vi "_Read_C.vi"(8 "error in (no error)":errorcluster, 11 "Postgres Connector In":refnum<class "Postgres Connector.lvclass">) -> (0 "error out":errorcluster, 1 "Another Query?":bool, 2 "No return?":bool, 3 "Postgres Connector Out":refnum<class "Postgres Connector.lvclass">)   [LabVIEW 2020, in "Postgres Connector.lvclass"]
doc: "This VI decode the \"C\" section of the message sent by the database. It also check if a another query has been sent. It return the type of query that has been completed"
uses:
  Postgres Connector.lvclass
  Cluster_Reader_Infos.ctl
  Enum_RowDescription_State_Machine.ctl
  Postgres Connector.lvclass/Postgres Connector.ctl
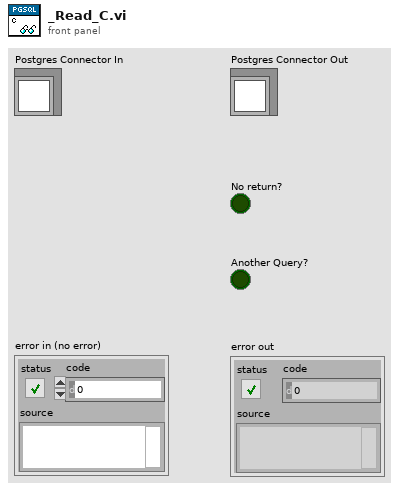
[diagram p1: front panel]
types:
  T1 = typedef "Postgres Connector.lvclass/Enum_RowDescription_State_Machine.ctl" = enum16{"Check For Error", "Wait For T", "Wait For D", "Wait For Z", "C Byte Length", "Z Byte Length", "n Byte Length", "Byte Length", "Get Infos", "Check For End", "Flush", "Quit"}
  T2 = typedef "Postgres Connector.lvclass/Cluster_Reader_Infos.ctl" = cluster{"Byte Length":i32}
  T3 = enum16{"Standard", "Buffered", "CRLF", "Immediate"}
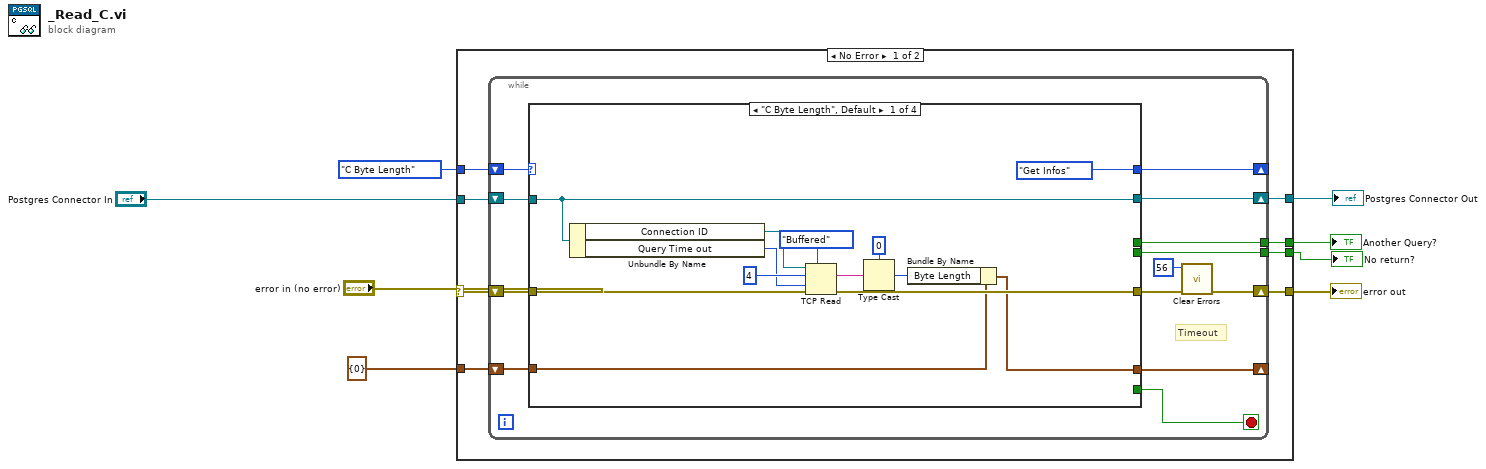
[diagram p0: block diagram]
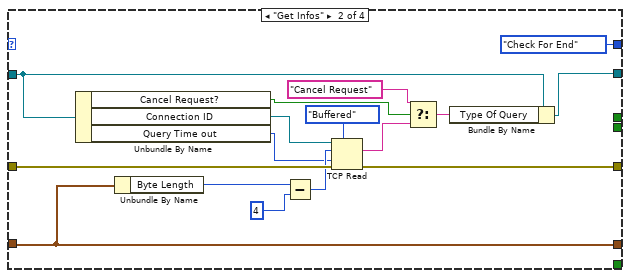
[diagram p2: hidden frame]
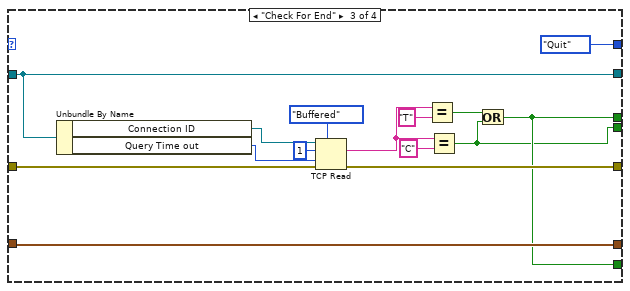
[diagram p3: hidden frame]
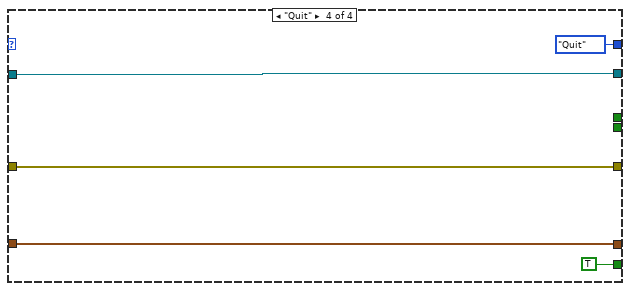
[diagram p4: hidden frame]
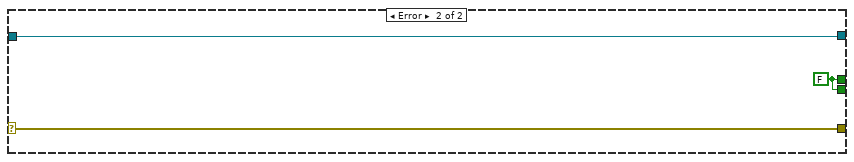
[diagram p5: hidden frame]
diagram:
  n1 = case shown="No Error" "error in (no error)" {
    selector: "error in (no error)" -> [w15 w81]
    tunnel: "Postgres Connector In" -> [w16 w80]
    tunnel: Enum_RowDescription_State_Machine."C Byte Length" -> [w14 _]
    tunnel: [w13 w81] -> w6
    tunnel: T2 {"Byte Length"=0} ("Reader_Infos") -> [w12 _]
    tunnel: [w11 w79] -> w4
    tunnel: [w10 w80] -> w3
    tunnel: [w9 w79] -> w2
    frame No Error {
      n2 = while {
        shift-right: [w25] -> w13
        shift-left: w15 -> [w28]
        shift-right: [w23] -> _
        shift-left: w14 -> [w27]
        shift-right: [w21] -> _
        shift-left: w12 -> [w22]
        tunnel: [w19] -> w11
        shift-right: [w18] -> w10
        shift-left: w16 -> [w29]
        tunnel: [w17] -> w9
        stop <- w20 stop-if-true
        # "Timeout"
        n3 = case shown="\"C Byte Length\", Default" w27 {
          tunnel: w29 -> [w38 w49 w65 w74]
          tunnel: w28 -> [w39 w56 w69 w77]
          tunnel: [w37 w55 w68 w77] -> w26
          tunnel: [Enum_RowDescription_State_Machine."Get Infos" Enum_RowDescription_State_Machine."Check For End" Enum_RowDescription_State_Machine."Quit" Enum_RowDescription_State_Machine."Quit"] -> w23
          tunnel: w22 -> [w36 w53 w67 w78]
          tunnel: [w35 w53 w67 w78] -> w21
          tunnel: [_ _ w62 TRUE] -> w20
          tunnel: [_ _ w62 _] -> w19
          tunnel: [w38 w48 w65 w74] -> w18
          tunnel: [_ _ w61 _] -> w17
          frame "C Byte Length", Default {
            n4 = Unbundle By Name(w38) -> ("Connection ID"=w41:refnum<k5>, "Query Time out"=w30:i32)
            n5 = TCP Read(connection ID=w41, bytes to read=4, error in (no error)=w39, 7:T3."Buffered" ("mode (standard)"), 9:w30) -> (data out=w31:string, error out=w37:errorcluster)  [unwired: 1 out]
            n6 = Type Cast(type=0, x=w31) -> (*(type *) &x=w32:i32)
            n7 = Bundle By Name(cluster=w36, "Byte Length"=w32) -> (w35:T2)
          }
          frame "Get Infos" {
            n8 = Unbundle By Name(w49) -> ("Cancel Request?"=w43:bool, "Connection ID"=w57:refnum<k5>, "Query Time out"=w47:i32)
            n9 = Unbundle By Name(w53) -> ("Byte Length"=w52:i32)
            n10 = Subtract(x=w52, y=4 ("bytes to read")) -> (x-y=w51:i32)
            n11 = TCP Read(connection ID=w57, bytes to read=w51, error in (no error)=w56, 7:T3."Buffered" ("mode (standard)"), 9:w47) -> (data out=w46:string, error out=w55:errorcluster)  [unwired: 1 out]
            n12 = Select(t="Cancel Request", s=w43, f=w46) -> (s? t:f=w45:string)
            n13 = Bundle By Name(cluster=w49, "Type Of Query"=w45) -> (w48:refnum<class "Postgres Connector.lvclass">)
          }
          frame "Check For End" {
            n14 = Unbundle By Name(w65) -> ("Connection ID"=w72:refnum<k5>, "Query Time out"=w59:i32)
            n15 = TCP Read(connection ID=w72, bytes to read=1, error in (no error)=w69, 7:T3."Buffered" ("mode (standard)"), 9:w59) -> (data out=w60:string, error out=w68:errorcluster)  [unwired: 1 out]
            n16 = Equal?(x=w60, y="T") -> (x = y?=w63:bool)
            n17 = Equal?(x=w60, y="C") -> (x = y?=w61:bool)
            n18 = Or(x=w63, y=w61) -> (x .or. y?=w62:bool)
          }
          frame "Quit" {
          }
        }
        n19 = call <vilib>:"Clear Errors.vi"("error in (no error)"=w26, "specific error code to clear (0: all)"=56) -> ("error out"=w25:errorcluster)  [unwired: 4 in, 1 out]
      }
    }
    frame Error {
      w79 = FALSE
    }
  }
  "error out" <- w6
  "Another Query?" <- w4
  "Postgres Connector Out" <- w3
  "No return?" <- w2
